vi "Find Center.vi"(5 "Position":i32, 7 "Tray Number":dbl format="%#_13g", 8 "Assembly Type":string, 9 "XYZTheta":dbl[](array[numeric]), 11 "Gantry In":refnum<k24>) -> (1 "XYZTheta Centers":dbl[][](array[numeric]), 3 "Gantry Out":refnum<k24>)   [LabVIEW 2021, in "Assembly Tray.lvclass"]
uses:
  Assembly Tray.lvclass
  Find Tray.ctl
  Controller/Camera/Machine Vision.ctl
  C:/Program Files (x86)/Aerotech/A3200/LabVIEW/2010/Bin/Aerotech.A3200.dll
  Program Files (x86)/Aerotech/A3200/LabVIEW/2010/Bin/Aerotech.A3200.dll
  Controller/Camera/Image processing.ctl
  Controller/Camera/Camera settings.ctl
  Controller/Camera/Material.ctl
  Controller/Camera/Camera.lvclass
  Controller/Motion/A3200/A3200.lvclass
  Controller/Motion/Motion.lvclass
panel:
  out "Low Speed":bool
  out "X":bool
  out "Y":bool
  out "Z":bool
  out "High Speed":bool
  out "Boolean 4":bool
  in  "Boolean 3":bool
  out "Move by":dbl[](array[numeric])
  in  "Autofiducial (Beta)":bool
  in  "Focus step size":dbl format="%#_13g"
  in  "number of focus steps":i32
  out "Average Strength":dbl
  in  "Focus":bool
  in  "Material":T1
  in  "Camera settings":T2={"Gamma"=1.6, "Gain"=0, "Sharpness"=0, "Contrast"=0.0, "Exposure"=0.0078125} {"Exposure" min=0.000244140625 max=0.5 scale=0.0002..0.5; "Contrast" min=0.0 max=1.0 scale=0.001..1.0; "Sharpness" min=0 max=2 step=1 scale=0.0..2.0; "Gain" min=0 max=100 step=1 scale=0.1..100.0; "Gamma" min=0.01 max=10.0 scale=0.01..10.0}
  in  "Image processing":T3={"Brightness"=128.0, "Contrast"=45.0, "Gamma"=1.0471123} {"Brightness" scale=0.0..400.0; "Contrast" scale=0.0..90.0; "Gamma" scale=0.005..5.0}
  in  "Override presets":bool
  out "Both fiducials recorded":bool
  in  "Machine Vision":T4
  out "Right Fiducial":dbl[](array[numeric]) format="%.6g"
  out "Left Fiducial":dbl[](array[numeric]) format="%.6g"
  out "Gantry":dbl[](array[numeric]) format="%.6g"
  out "Sum":dbl[](array[numeric]) format="%.6g"
  out "Camera":dbl[](array[numeric]) format="%.6g"
  in  "Carrier Tray":T5
  out "Image":T6(plugin-control)
  out "Center":dbl[](array[numeric]) format="%.6g"
  in  "Position Number":i16
  in  "Go to Center":bool
  in  "Calculate":bool
  in  "Record Bottom":bool
  in  "Record Top":bool
  in  "Go to Bottom Fiducial":bool
  in  "Go to Top Fiducial":bool
  in  "Joystick":bool
  in  "Stop":bool
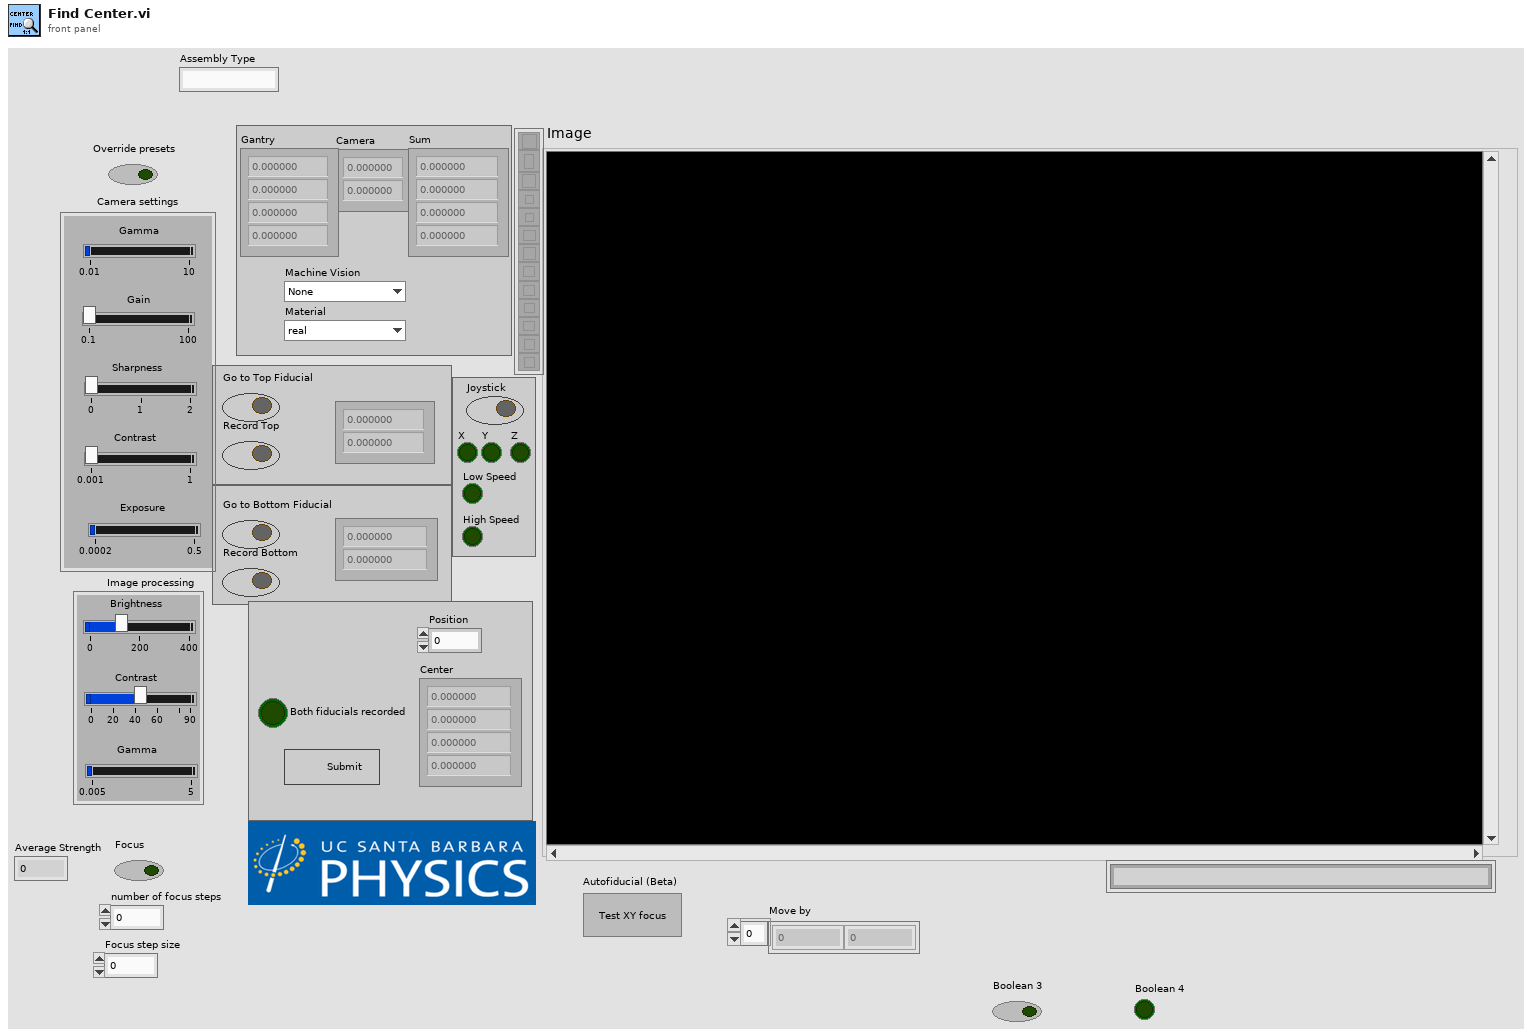
[diagram p1: front panel]
types:
  T1 = typedef "Camera.lvclass/Material.ctl" = enum16{"real", "dummy", "PETG"}
  T2 = typedef "Camera.lvclass/Camera settings.ctl" = cluster{"Gamma":dbl, "Gain":i64, "Sharpness":i64, "Contrast":dbl, "Exposure":dbl}
  T3 = typedef "Camera.lvclass/Image processing.ctl" = cluster{"Brightness":sgl, "Contrast":sgl, "Gamma":sgl}
  T4 = typedef "Camera.lvclass/Machine Vision.ctl" = enum16{"None", "Tray Fiducials", "Sensor Fiducials", "HPK Silicon", "Partial Hexaboard", "Partial Hexaboard Test", "100um dot", "Hexaboard", "Corner (TL, BR)", "Corner (BL, TR)", "V3 Sensor Cross", "V3 Sensor Circle", "test"}
  T5 = typedef "Assembly Tray.lvclass/Find Tray.ctl" = cluster{"Gantry Fiducials":dbl[], "Relative Coordinates":dbl[][], "Camera Fiducials":dbl[][], "XYZTheta Centers":dbl[][], "Workspace Center":dbl[], "Syringe Relative Coordinates":dbl[], "Gantry Region":dbl, "Fiducials":path, "New Fiducials":dbl[][], "Past Fiducials":dbl[][], "XYZTheta":dbl[]}
  T6 = typedef "IMAQ Image.ctl" = refnum<image>
  T7 = typedef "File Paths.ctl" = cluster{"Glue Pattern Folder":path, "Carrier Tray Folder":path, "Pick Up Tool Fixture Folder":path, "Components Folder":path, "Bellows Tool Offset.txt":path, "Pick Up Tool Offset.txt":path, "Dispense Tip Offset.txt":path, "Log Files":path, "Gantry Assembly Map.txt":path, "Syringe and offset map.txt":path, "Controllers Folder":path, "Local dbase config":path}
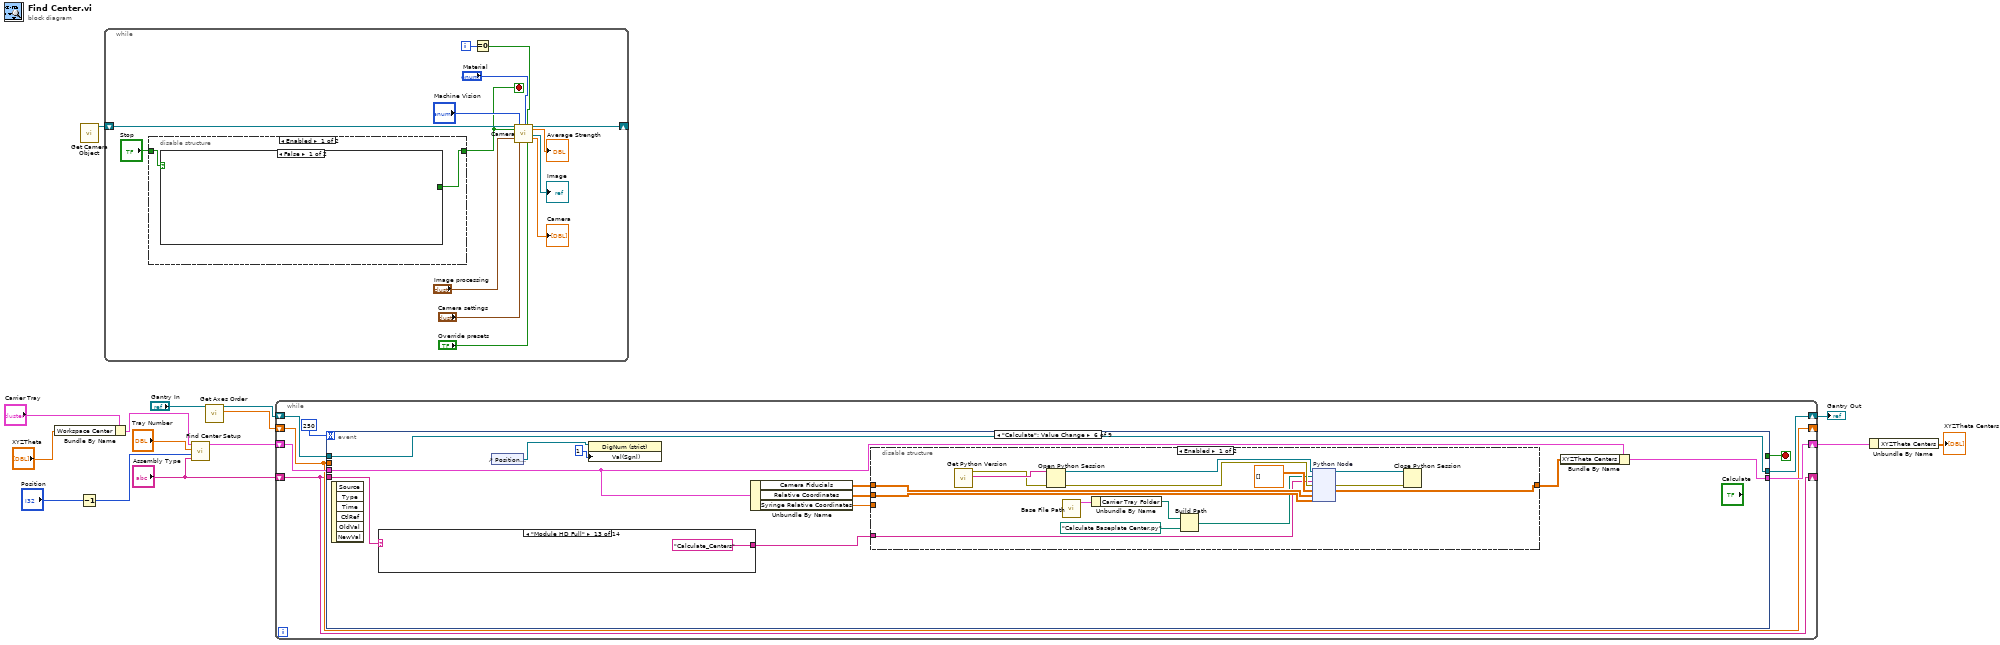
[diagram p0: block diagram]
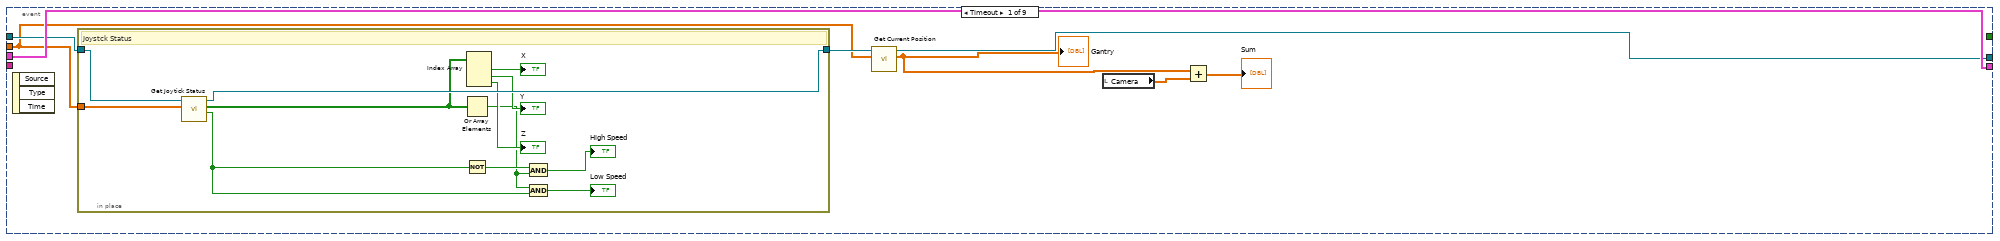
[diagram p2: hidden frame]
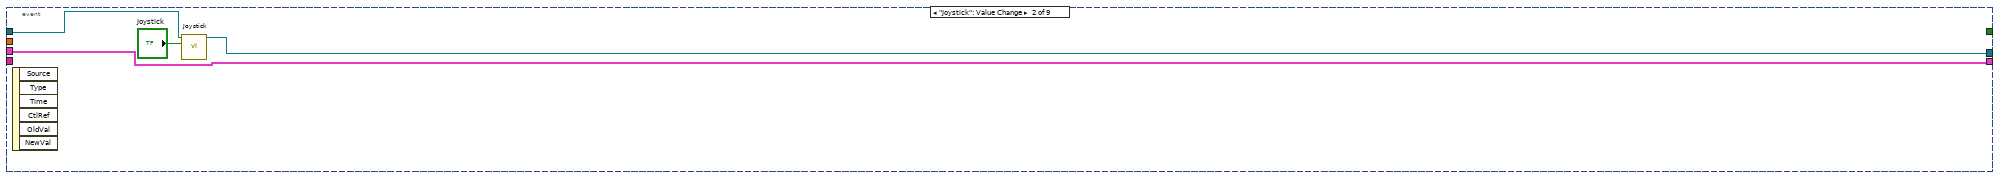
[diagram p3: hidden frame]
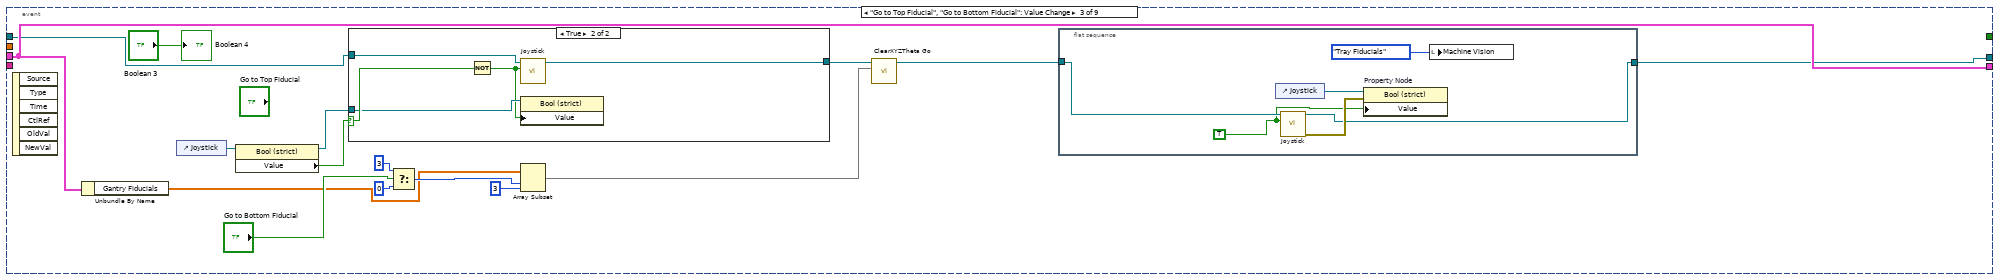
[diagram p4: hidden frame]
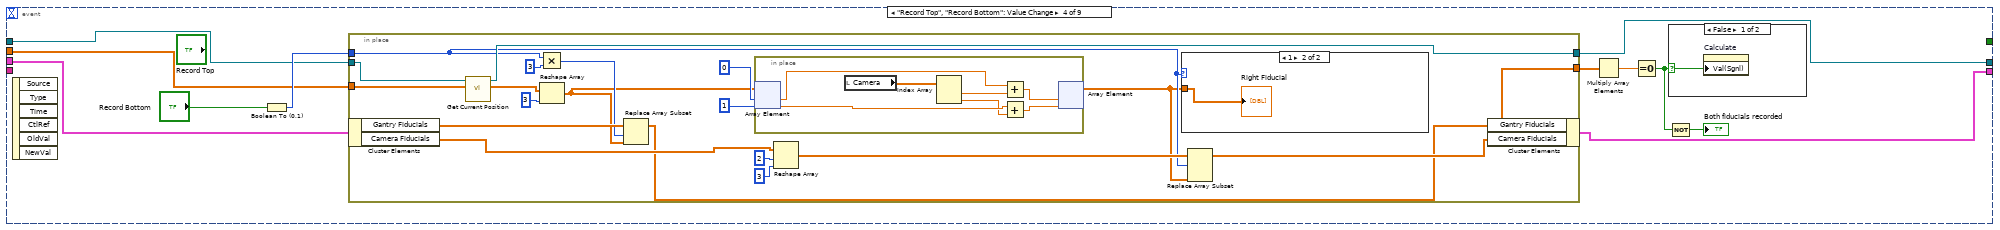
[diagram p6: hidden frame]
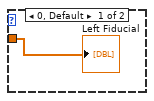
[diagram p8: hidden frame]
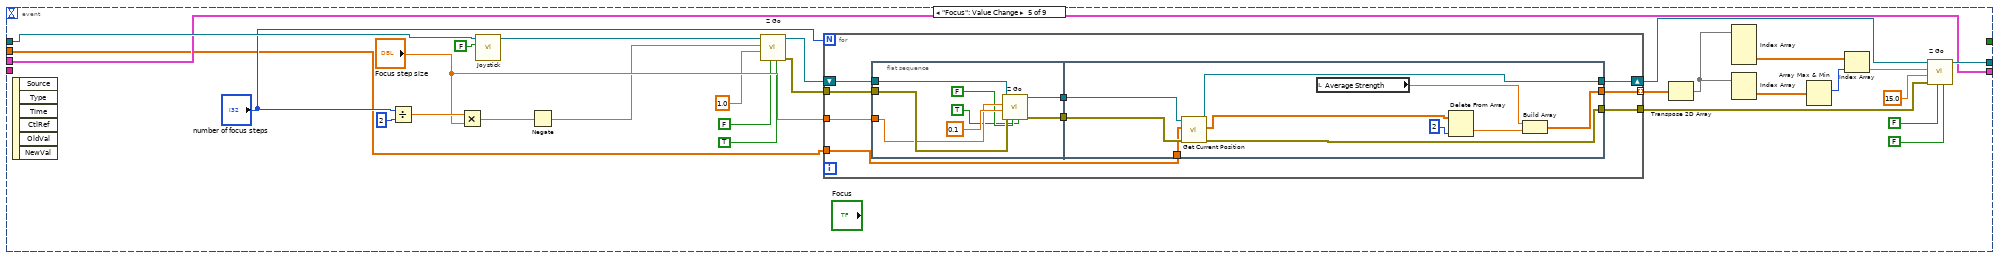
[diagram p9: hidden frame]
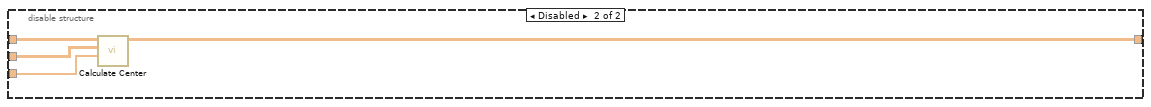
[diagram p10: hidden frame]
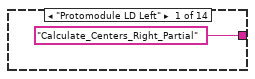
[diagram p11: hidden frame]
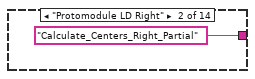
[diagram p12: hidden frame]
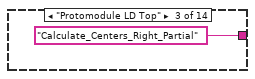
[diagram p13: hidden frame]
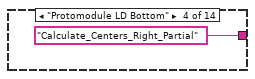
[diagram p14: hidden frame]
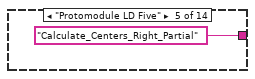
[diagram p15: hidden frame]
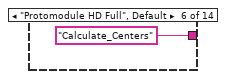
[diagram p16: hidden frame]
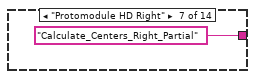
[diagram p17: hidden frame]
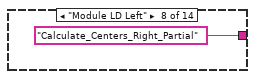
[diagram p18: hidden frame]
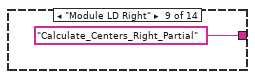
[diagram p19: hidden frame]
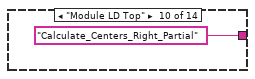
[diagram p20: hidden frame]
diagram:
  n1 = Bundle By Name(cluster="Carrier Tray", "Workspace Center"="XYZTheta") -> (w12:T5)
  n2 = call "Get Camera Object.vi"() -> ("Camera out"=w8:refnum<class "Camera.lvclass">)  [unwired: 10 in, 1 out]
  n3 = Decrement(x="Position") -> (x-1=w6:i32)
  n4 = while {
    shift-right: [w25] -> _
    shift-left: w8 -> [w29]
    i -> [w19]
    stop <- w24 stop-if-true
    n5 = disable-structure shown="Enabled" {
      disable-tunnel: [w30 w37] -> w24
      disable-tunnel: "Stop" -> [w31 w37]
      frame Enabled {
        n6 = case shown="False" w31 {
          tunnel: [_ w32] -> w30
          frame False {
          }
          frame True {
            n7 = property on="Both fiducials recorded" class="Bool (strict)"() -> ("Value"=w33:bool)  [unwired: 2 in, 2 out]
            n8 = case shown="False" w33 {
              tunnel: [_ TRUE] -> w32
              frame False {
                n9 = One Button Dialog(message="Atleast one fiducial not recorded!") -> ()  [unwired: 1 in, 1 out]
              }
              frame True {
                n10 = property on="Both fiducials recorded" class="Bool (strict)"("Val(Sgnl)"=FALSE) -> ()  [unwired: 2 in, 2 out]
              }
            }
          }
        }
      }
      frame Disabled {
      }
    }
    n11 = Equal To 0?(x=w19) -> (x = 0?=w18:bool)
    n12 = call "Camera.vi"("Camera in"=w29, "Stop"=w24, "BCG Image Processing"="Image processing", "Machine Vision"="Machine Vision", "Camera settings"="Camera settings", "Material"="Material", "Loop 0"=w18, "Override presets"="Override presets") -> ("Camera out"=w25:refnum<class "Camera.lvclass">, "Average Strength"=→"Average Strength":dbl, "Image"=→"Image":T6, "Camera"=→"Camera":dbl[])  [unwired: 5 in, 3 out]
  }
  n13 = call "Find Center Setup.vi"("Carrier Tray"=w12, "Tray Number"="Tray Number", "Position"=w6, "Assembly Type"="Assembly Type") -> ("Assembly Tray Out"=w15:T5)  [unwired: 6 in]
  n14 = call "Get Axes Order.vi"("Gantry In"="Gantry In") -> ("Axes Order"=w2:dbl[], "Gantry Out"=w3:refnum<k24>)  [unwired: 8 in, 1 out]
  n15 = while {
    shift-right: [w44] -> w14
    shift-left: w15 -> [w45]
    shift-right: [w40] -> w7
    shift-left: w3 -> [w41]
    shift-right: [w39] -> _
    shift-left: w2 -> [w39]
    shift-right: [w38] -> _
    shift-left: "Assembly Type" -> [w38]
    stop <- w43 stop-if-true
    n16 = event shown="[5] \"Calculate\": Value Change" {
      selector: _ -> [_ _ _ _ _ _ _ _ _]
      dyn-events: _ -> [_ _ _ _ _ _ _ _ _]
      timeout: 250 -> [_ _ _ _ _ _ _ _ _]
      tunnel: [w51 w69 w85 w108 w150 w195 w246 w273 w286] -> w44
      tunnel: w45 -> [w51 w69 w85 w103 w150 w196 w247 w273 w286]
      tunnel: [_ _ _ _ _ _ _ w268 _] -> w43
      tunnel: w41 -> [w48 w68 w77 w102 w152 w201 w244 w274 w288]
      tunnel: [w49 w66 w72 w101 w151 w201 w241 w269 w289] -> w40
      tunnel: w38 -> [_ _ _ _ _ w197 _ _ _]
      tunnel: w39 -> [w46 _ _ w98 w138 _ _ _ _]
      event Timeout {
        n17 = event-data() -> ()  [unwired: 1 in, 3 out]
        n18 = in-place {
          in-place-border: w48 -> [w65]
          in-place-border: [w64] -> w47
          in-place-border: w46 -> [w63]
          # "Joystck Status"
          n19 = call "Get Joytick Status.vi"("Axes Order"=w63, "Gantry In"=w65) -> ("JoystickLowSpeedActive"=w57:bool, "Joystick Status"=w59:bool[], "Gantry Out"=w64:refnum<k24>)  [unwired: 6 in, 1 out]
          n20 = Or Array Elements(Boolean array=w59) -> (logical OR=w55:bool)
          n21 = Not(x=w57) -> (.not. x?=w56:bool)
          n22 = Index Array(array=w59) -> (element #1=→"X":bool, element #2=→"Y":bool, element #3=→"Z":bool)  [unwired: 3 in]
          n23 = And(x=w56, y=w55) -> (x .and. y?=→"High Speed":bool)
          n24 = And(x=w55, y=w57) -> (x .and. y?=→"Low Speed":bool)
        }
        n25 = call "Get Current Position.vi"("Axes Order"=w46, "Gantry In"=w47) -> ("XYZTheta Out"=w50:dbl[], "Gantry Out"=w49:refnum<k24>)  [unwired: 7 in, 1 out]
        "Gantry" <- w50
        n26 = local read "Camera"() -> (w53:dbl[])
        n27 = Add(x=w50, y=w53) -> (x+y=→"Sum":dbl[])
      }
      event "Joystick": Value Change {
        n28 = event-data() -> ()  [unwired: 1 in, 6 out]
        n29 = call "Joystick.vi"("Joystick"="Joystick", "Gantry In"=w68) -> ("Gantry Out"=w66:refnum<k24>)  [unwired: 8 in, 1 out]
      }
      event "Go to Top Fiducial", "Go to Bottom Fiducial": Value Change {
        n30 = event-data() -> ()  [unwired: 1 in, 6 out]
        n31 = Unbundle By Name "Unbundle By Name"(w85) -> ("Gantry Fiducials"=w74:dbl[])
        n32 = control-ref of="Joystick"() -> (w84:refnum<vi>)
        n33 = property class="Bool (strict)"(reference=w84) -> (reference out=w75:refnum<vi>, "Value"=w78:bool)  [unwired: 1 in, 1 out]
        n34 = case shown="True" w78 {
          selector: w78 -> [_ w97]
          tunnel: w77 -> [w92 w95]
          tunnel: [w92 w94] -> w76
          tunnel: w75 -> [_ w96]
          frame False {
          }
          frame True {
            n35 = Not(x=w97) -> (.not. x?=w93:bool)
            n36 = call "Joystick.vi"("Joystick"=w93, "Gantry In"=w95) -> ("Gantry Out"=w94:refnum<k24>)  [unwired: 8 in, 1 out]
            n37 = property class="Bool (strict)"(reference=w96, "Value"=w93) -> ()  [unwired: 1 in, 2 out]
          }
        }
        n38 = Select(t=3, s="Go to Bottom Fiducial", f=0) -> (s? t:f=w82:i32)
        n39 = Array Subset "Array Subset"(array=w74, index=w82, length=3) -> (w73:dbl[])
        n40 = call "ClearXYZTheta Go.vi"("XYZTheta In"=w73, "Gantry In"=w76) -> ("Gantry Out"=w71:refnum<k24>)  [unwired: 7 in, 2 out]
        n41 = flat-sequence {
          tunnel: w71 -> [w91]
          tunnel: [w88] -> w72
          frame #0 {
            w87 = TRUE
            n42 = control-ref of="Joystick"() -> (w90:refnum<vi>)
            n43 = call "Joystick.vi"("Joystick"=w87, "Gantry In"=w91) -> ("error out"=w89:errorcluster, "Gantry Out"=w88:refnum<k24>)  [unwired: 8 in]
            n44 = property on="Property Node" class="Bool (strict)"(reference=w90, error in=w89, "Value"=w87) -> ()  [unwired: 2 out]
            n45 = local write "Machine Vision"(Machine_Vision."Tray Fiducials" ("Machine Vision")) -> ()
          }
        }
        "Boolean 4" <- "Boolean 3"
      }
      event "Record Top", "Record Bottom": Value Change {
        n46 = event-data() -> ()  [unwired: 1 in, 6 out]
        n47 = Boolean To (0,1)(Boolean="Record Bottom") -> (0, 1=w105:i16)
        n48 = in-place {
          in-place-border: [w122] -> w106
          in-place-border: w105 -> [w115]
          in-place-border: w102 -> [w117]
          in-place-border: [w116] -> w101
          in-place-border: w98 -> [w110]
          n49 = in-place-cluster #1(w103) -> ("Gantry Fiducials"=w119:dbl[], "Camera Fiducials"=w126:dbl[][])
          n50 = call "Get Current Position.vi"("Axes Order"=w110, "Gantry In"=w117) -> ("XYZTheta Out"=w120:dbl[], "Gantry Out"=w116:refnum<k24>)  [unwired: 7 in, 1 out]
          n51 = Multiply(x=w115, y=i16 3) -> (x*y=w113:i16)
          n52 = Reshape Array(w120, 3 ("dimension size")) -> (w112:dbl[])
          n53 = Replace Array Subset(array=w119, new element=w112, index=w113) -> (w118:dbl[])
          n54 = in-place {
            n55 = in-place-array #2(w112, 0, 1) -> (w134:dbl, w132:dbl)
            n56 = local read "Camera"() -> (w135:dbl[])
            n57 = Index Array(array=w135) -> (element #1=w133:dbl, element #2=w131:dbl)  [unwired: 2 in]
            n58 = Add(x=w134, y=w133) -> (x+y=w129:dbl)
            n59 = Add(x=w132, y=w131) -> (x+y=w130:dbl)
            n60 = in-place-array #2(w129, w130) -> (w111:dbl[])  [unwired: 2 out]
          }
          n61 = Reshape Array(w126, 2 ("length"), 3 ("dimension size")) -> (w125:dbl[][])
          n62 = case shown="1" w115 {
            tunnel: w111 -> [w136 w137]
            frame 0, Default {
              "Left Fiducial" <- w136
            }
            frame 1 {
              "Right Fiducial" <- w137
            }
          }
          n63 = Replace Array Subset(array=w125, new element=w111, index (row)=w115) -> (w122:dbl[][])  [unwired: 1 in]
          n64 = in-place-cluster #1("Gantry Fiducials"=w118, "Camera Fiducials"=w122) -> (w108:T5)
        }
        n65 = Multiply Array Elements(1:w106) -> (0:w107:dbl)
        n66 = Equal To 0?(x=w107) -> (x = 0?=w100:bool)
        n67 = Not(x=w100) -> (.not. x?=→"Both fiducials recorded":bool)
        n68 = case shown="False" w100 {
          selector: w100 -> [w109 _]
          frame False {
            n69 = property on="Calculate" class="Bool (strict)"("Val(Sgnl)"=w109) -> ()  [unwired: 2 in, 2 out]
          }
          frame True {
          }
        }
      }
      event "Focus": Value Change {
        n70 = event-data() -> ()  [unwired: 1 in, 6 out]
        n71 = Divide(x="number of focus steps", y=2) -> (x/y=w154:dbl)
        n72 = Multiply(x=w154, y="Focus step size") -> (x*y=w153:dbl)
        n73 = call "Joystick.vi"("Joystick"=FALSE, "Gantry In"=w152) -> ("Gantry Out"=w146:refnum<k24>)  [unwired: 8 in, 1 out]
        n74 = Negate(x=w153) -> (-x=w144:dbl)
        n75 = call "Z Go.vi"("Increment"=TRUE, "Return Immediately"=FALSE ("Increment"), "Speed In"=1.0 ("Speed"), "Position In"=w144, "Gantry In"=w146) -> ("error out"=w141:errorcluster, "Gantry Out"=w145:refnum<k24>)  [unwired: 3 in, 2 out]
        n76 = for {
          N: "number of focus steps" -> [_]
          tunnel: [w171] -> w164 mode=indexing
          tunnel: w141 -> [w170]
          tunnel: [w168] -> w157
          shift-right: [w172] -> w158
          shift-left: w145 -> [w174]
          tunnel: "Focus step size" -> [w167]
          tunnel: w138 -> [w166]
          n77 = flat-sequence {
            tunnel: w174 -> [w182]
            tunnel: [w181] -> w173
            tunnel: w170 -> [w179]
            tunnel: [w180] -> w169
            tunnel: w167 -> [w177]
            tunnel: w173 -> [w192]
            tunnel: [w191] -> w172
            tunnel: [w190] -> w171
            tunnel: w169 -> [w186]
            tunnel: [w185] -> w168
            tunnel: w166 -> [w183]
            frame #0 {
              n78 = call "Z Go.vi"("Increment"=TRUE, "Return Immediately"=FALSE ("Increment"), "error in (no error)"=w179, "Speed In"=0.1 ("Speed"), "Position In"=w177, "Gantry In"=w182) -> ("error out"=w180:errorcluster, "Gantry Out"=w181:refnum<k24>)  [unwired: 2 in, 2 out]
            }
            frame #1 {
              n79 = call "Get Current Position.vi"("error in (no error)"=w186, "Axes Order"=w183, "Gantry In"=w192) -> ("error out"=w185:errorcluster, "XYZTheta Out"=w189:dbl[], "Gantry Out"=w191:refnum<k24>)  [unwired: 6 in]
              n80 = local read "Average Strength"() -> (w184:dbl)
              n81 = Delete From Array(array=w189, index=2) -> (deleted portion=w187:dbl)  [unwired: 1 in, 1 out]
              n82 = Build Array(w184, w187) -> (w190:dbl[])
            }
          }
        }
        n83 = Transpose 2D Array(2D array=w164) -> (transposed array=w163:dbl[][])
        n84 = Index Array(array=w163) -> (element #2=w162:dbl[])  [unwired: 4 in, 1 out]
        n85 = Index Array(array=w163) -> (element=w165:dbl[])  [unwired: 2 in]
        n86 = Array Max & Min(array=w165) -> (max index (indices)=w161:i32)  [unwired: 3 out]
        n87 = Index Array(array=w162, index=w161) -> (element=w160:dbl)
        n88 = call "Z Go.vi"("Increment"=FALSE, "Return Immediately"=FALSE ("Increment"), "error in (no error)"=w157, "Speed In"=15.0 ("Speed"), "Position In"=w160, "Gantry In"=w158) -> ("Gantry Out"=w151:refnum<k24>)  [unwired: 2 in, 3 out]
      }
      event "Calculate": Value Change {
        n89 = event-data() -> ()  [unwired: 1 in, 6 out]
        n90 = case shown="\"Module HD Full\"" w197 {
          tunnel: ["Calculate_Centers_Right_Partial" ("function name") "Calculate_Centers_Right_Partial" ("function name") "Calculate_Centers_Right_Partial" ("function name") "Calculate_Centers_Right_Partial" ("function name") "Calculate_Centers_Right_Partial" ("function name") "Calculate_Centers" ("function name") "Calculate_Centers_Right_Partial" ("function name") "Calculate_Centers_Right_Partial" ("function name") "Calculate_Centers_Right_Partial" ("function name") "Calculate_Centers_Right_Partial" ("function name") "Calculate_Centers_Right_Partial" ("function name") "Calculate_Centers_Right_Partial" ("function name") "Calculate_Centers" ("function name") "Calculate_Centers_Right_Partial" ("function name")] -> w194
          frame "Protomodule LD Left" {
          }
          frame "Protomodule LD Right" {
          }
          frame "Protomodule LD Top" {
          }
          frame "Protomodule LD Bottom" {
          }
          frame "Protomodule LD Five" {
          }
          frame "Protomodule HD Full", Default {
          }
          frame "Protomodule HD Right" {
          }
          frame "Module LD Left" {
          }
          frame "Module LD Right" {
          }
          frame "Module LD Top" {
          }
          frame "Module LD Bottom" {
          }
          frame "Module LD Five" {
          }
          frame "Module HD Full" {
          }
          frame "Module HD Right" {
          }
        }
        n91 = control-ref of="Position Number"() -> (w203:refnum<vi>)
        n92 = property class="DigNum (strict)"(reference=w203, "Val(Sgnl)"=i16 1 ("Value (Signaling)")) -> ()  [unwired: 1 in, 2 out]
        n93 = Unbundle By Name "Unbundle By Name"(w196) -> ("Camera Fiducials"=w198:dbl[][], "Relative Coordinates"=w199:dbl[][], "Syringe Relative Coordinates"=w200:dbl[])
        n94 = disable-structure shown="Enabled" {
          disable-tunnel: w198 -> [w213 w221]
          disable-tunnel: w199 -> [w212 w220]
          disable-tunnel: w200 -> [_ w219]
          disable-tunnel: [w207 w222] -> w193
          disable-tunnel: w194 -> [w206 _]
          frame Enabled {
            n95 = call "Get Python Version.vi"() -> ("Python Version"=w205:string, "error out"=w204:errorcluster)  [unwired: 10 in]
            n96 = Open Python Session(python version=w205, 3:w204) -> (session out=w218:refnum<k35>, error out=w216:errorcluster)  [unwired: 1 in]
            n97 = call "Base File Path.vi"() -> ("Paths Out"=w214:T7)  [unwired: 11 in]
            n98 = Unbundle By Name(w214) -> ("Carrier Tray Folder"=w210:path)
            n99 = Build Path(base path=w210, name or relative path=path "Calculate Baseplate Center.py") -> (appended path=w209:path)
            n100 = node "Python Node"(w218, w209, w206, w216, dbl[][] [], w213, w212) -> (w217:refnum<k35>, w215:errorcluster, w207:dbl[][])  [unwired: 2 in, 2 out]
            n101 = Close Python Session(session in=w217, error in=w215) -> ()  [unwired: 1 out]
          }
          frame Disabled {
            n102 = call "Calculate Center.vi"("Syringe Coordinates"=w219, "Relative Coordinates"=w220, "Fiducial Measurements"=w221) -> ("XYZTheta Centers"=w222:dbl[][])  [unwired: 8 in]
          }
        }
        n103 = Bundle By Name(cluster=w196, "XYZTheta Centers"=w193) -> (w195:T5)
      }
      event "Go to Center", "Position Number": Value Change {
        n104 = event-data() -> ()  [unwired: 1 in, 6 out]
        n105 = disable-structure shown="Enabled" {
          disable-tunnel: ["Position Number" _] -> w238
          frame Enabled {
          }
          frame Disabled {
          }
        }
        n106 = Unbundle By Name(w247) -> ("XYZTheta Centers"=w240:dbl[][])
        n107 = Decrement(x=w238) -> (x-1=w239:i16)
        n108 = Index Array "Index Array"(array=w240, index (row)=w239) -> (element=w242:dbl[])  [unwired: 1 in]
        n109 = Reshape Array "Reshape Array"(w242, u32 4) -> (w237:dbl[])
        n110 = case shown="False" "Go to Center" {
          tunnel: w237 -> [w249 w257]
          tunnel: w247 -> [w251 w259]
          tunnel: [w251 w259] -> w246
          tunnel: w244 -> [w250 w253]
          tunnel: [w250 w258] -> w241
          frame False {
            # "Change Position Number"
            "Center" <- w249
          }
          frame True {
            n111 = control-ref of="Joystick"() -> (w256:refnum<vi>)
            n112 = property class="Bool (strict)"(reference=w256) -> (reference out=w254:refnum<vi>, "Value"=w255:bool)  [unwired: 1 in, 1 out]
            n113 = case shown="True" w255 {
              selector: w255 -> [_ w265]
              tunnel: w253 -> [w260 w264]
              tunnel: [w260 w263] -> w252
              tunnel: w254 -> [_ w261]
              frame False {
              }
              frame True {
                n114 = Not(x=w265) -> (.not. x?=w262:bool)
                n115 = property class="Bool (strict)"(reference=w261, "Value"=w262) -> ()  [unwired: 1 in, 2 out]
                n116 = call "Joystick.vi"("Joystick"=w262, "Gantry In"=w264) -> ("Gantry Out"=w263:refnum<k24>)  [unwired: 8 in, 1 out]
              }
            }
            n117 = call "ClearXYZTheta Go.vi"("XYZTheta In"=w257, "Gantry In"=w252) -> ("Gantry Out"=w258:refnum<k24>)  [unwired: 7 in, 2 out]
          }
        }
      }
      event "Stop": Value Change {
        n118 = event-data() -> ()  [unwired: 1 in, 6 out]
        n119 = Unbundle By Name(w273) -> ("Fiducials"=w271:path, "Gantry Fiducials"=w272:dbl[])
        n120 = call "Replace Row In File.vi"("Index"=0, "Insert Array"=w272, "Path"=w271) -> ("error out"=w277:errorcluster)  [unwired: 8 in]
        n121 = property on="Both fiducials recorded" class="Bool (strict)"() -> ("Value"=w266:bool)  [unwired: 2 in, 2 out]
        n122 = case shown="No Error" w277 {
          tunnel: "Fiducial" -> [w278 w285]
          frame No Error {
            w279 = "\r"
            n123 = Concatenate Strings("Success!", w279, w279, w278, " Values Stored") -> ()  [unwired: 1 out]
          }
          frame Error {
            w282 = "\r"
            n124 = Concatenate Strings("Error!", w282, w282, w285, " Values Not Stored") -> ()  [unwired: 1 out]
          }
        }
        n125 = And(x=w266, y=TRUE) -> (x .and. y?=w268:bool)
        n126 = call "Joystick.vi"("Joystick"=FALSE, "Gantry In"=w274) -> ("Gantry Out"=w269:refnum<k24>)  [unwired: 8 in, 1 out]
      }
      event "Autofiducial (Beta)": Value Change {
        n127 = event-data() -> ()  [unwired: 1 in, 6 out]
        n128 = disable-structure shown="Enabled" {
          disable-tunnel: [w293 w320] -> w289
          disable-tunnel: w288 -> [w292 w320]
          disable-tunnel: "Autofiducial (Beta)" -> [w291 _]
          frame Enabled {
            n129 = flat-sequence {
              tunnel: w291 -> [_]
              tunnel: [w299] -> w290
              tunnel: w292 -> [w304]
              tunnel: [w304] -> w298
              tunnel: [w303] -> w297
              tunnel: [w302] -> w296
              tunnel: w290 -> [w301]
              tunnel: w298 -> [w308]
              tunnel: [w307] -> w295
              tunnel: w297 -> [w306]
              tunnel: [w305] -> w294
              tunnel: w296 -> [w305]
              tunnel: [w314] -> w293
              tunnel: w295 -> [w315]
              tunnel: w294 -> [w313]
              frame #0 {
                n130 = local read "Image"() -> (w300:T6)
                n131 = call "Find Fiducial.vi"("Image"=w300) -> ("Move by (mm)"=w299:dbl[])  [unwired: 3 in]
              }
              frame #1 {
                n132 = Index Array(array=w301) -> (element #1=w303:dbl, element #2=w302:dbl)  [unwired: 2 in]
                "Move by" <- w301
              }
              frame #2 {
                n133 = call "Joystick.vi"("Joystick"=FALSE, "Gantry In"=w308) -> ("Gantry Out"=w309:refnum<k24>)  [unwired: 8 in, 1 out]
                n134 = call "Move Inc.vi"("Axis"="X", "Speed"=25.0, "Distance"=w306, "Gantry In"=w309) -> ("Gantry Out"=w307:refnum<k24>)  [unwired: 6 in, 1 out]
              }
              frame #3 {
                n135 = call "Joystick.vi"("Joystick"=FALSE, "Gantry In"=w315) -> ("Gantry Out"=w316:refnum<k24>)  [unwired: 8 in, 1 out]
                n136 = call "Move Inc.vi"("Axis"="Y", "Speed"=25.0, "Distance"=w313, "Gantry In"=w316) -> ("Gantry Out"=w314:refnum<k24>)  [unwired: 6 in, 1 out]
              }
            }
          }
          frame Disabled {
          }
        }
      }
    }
  }
  "Gantry Out" <- w7
  n137 = Unbundle By Name(w14) -> ("XYZTheta Centers"=→"XYZTheta Centers":dbl[][])
